vi "Adjust Color.vi"(1 "Greyscale In":u8) -> (0 "Greyscale Out":u8)   [LabVIEW 2016]
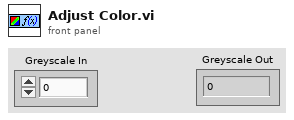
[diagram p1: front panel]
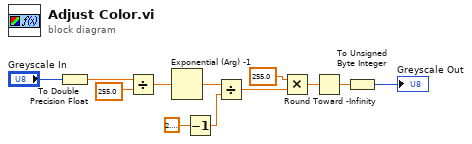
[diagram p0: block diagram]
diagram:
  n1 = To Double Precision Float(number="Greyscale In") -> (double precision float=w5:dbl)
  n2 = Divide(x=w5, y=255.0) -> (x/y=w11:dbl)
  n3 = Exponential (Arg) -1(1:w11) -> (0:w7:dbl)
  n4 = Decrement(x=2.718281828459045) -> (x-1=w6:dbl)
  n5 = Divide(x=w7, y=w6) -> (x/y=w8:dbl)
  n6 = Multiply(x=255.0 ("y"), y=w8) -> (x*y=w1:dbl)
  n7 = Round Toward -Infinity(1:w1) -> (0:w4:dbl)
  n8 = To Unsigned Byte Integer(number=w4) -> (unsigned 8bit integer=→"Greyscale Out":u8)
